vi "SwerveChooseBestAngle.vi"(5 "Goal Override":bool, 7 "Goal Override Angle (deg) [-180,+180]":dbl format="%#_13g", 8 "Hysteresis (deg)":dbl=10.0 format="%#_13g", 10 "Goal Angle (deg) [-180,+180]":dbl format="%#_13g", 11 "Current Angle (deg) [-180,+180]":dbl format="%#_13g") -> (0 "Flip Drive Motor Multiple":dbl, 2 "Angular Distance (deg)":dbl format="%_4g")   [LabVIEW 2020]
doc: "Based on the Current Angle and the Goal Angle, this VI calulates the signed angular distance. Taking into account the option to invert the direction of the swerve drive motor and always picking the shortest travel distance. The hysteresis prevents undesirable vacillation between angle choices."
panel:
  out "Flip Drive Motor Direction":bool
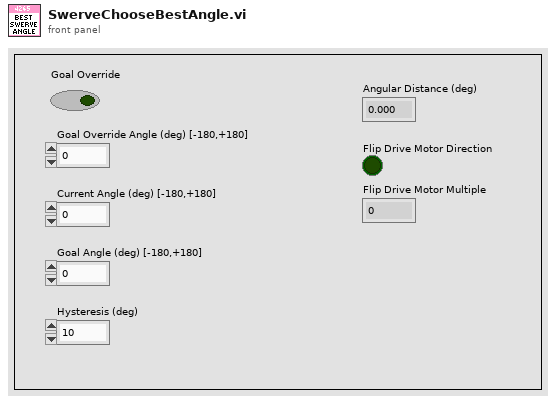
[diagram p1: front panel]
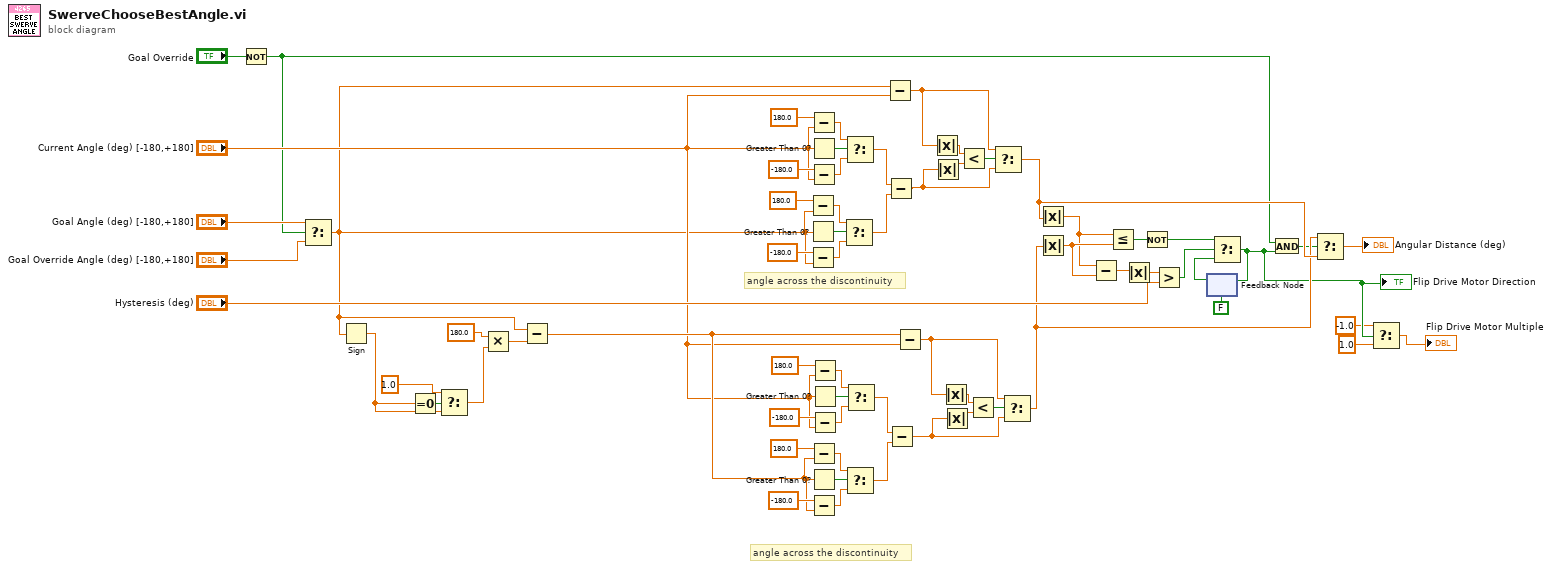
[diagram p0: block diagram]
diagram:
  # "angle across the discontinuity"
  # "angle across the discontinuity"
  n1 = Not(x="Goal Override") -> (.not. x?=w6:bool)
  n2 = Select(t="Goal Angle (deg) [-180,+180]", s=w6, f="Goal Override Angle (deg) [-180,+180]") -> (s? t:f=w8:dbl)
  n3 = Sign(1:w8) -> (0:w16:dbl)
  n4 = Equal To 0?(x=w16) -> (x = 0?=w17:bool)
  n5 = Select(t=1.0, s=w17, f=w16) -> (s? t:f=w13:dbl)
  n6 = Multiply(x=180.0 ("y"), y=w13) -> (x*y=w65:dbl)
  n7 = Subtract(x=w8, y=w65) -> (x-y=w38:dbl)
  n8 = Subtract(x=180.0, y=w8) -> (x-y=w26:dbl)
  n9 = Greater Than 0?(x=w8) -> (x > 0?=w28:bool)
  n10 = Subtract(x=-180.0, y=w8) -> (x-y=w24:dbl)
  n11 = Subtract(x=180.0, y="Current Angle (deg) [-180,+180]") -> (x-y=w31:dbl)
  n12 = Greater Than 0?(x="Current Angle (deg) [-180,+180]") -> (x > 0?=w33:bool)
  n13 = Subtract(x=-180.0, y="Current Angle (deg) [-180,+180]") -> (x-y=w29:dbl)
  n14 = Subtract(x=180.0, y=w38) -> (x-y=w47:dbl)
  n15 = Greater Than 0?(x=w38) -> (x > 0?=w49:bool)
  n16 = Subtract(x=-180.0, y=w38) -> (x-y=w45:dbl)
  n17 = Subtract(x=180.0, y="Current Angle (deg) [-180,+180]") -> (x-y=w53:dbl)
  n18 = Greater Than 0?(x="Current Angle (deg) [-180,+180]") -> (x > 0?=w55:bool)
  n19 = Subtract(x=-180.0, y="Current Angle (deg) [-180,+180]") -> (x-y=w51:dbl)
  n20 = Select(t=w26, s=w28, f=w24) -> (s? t:f=w22:dbl)
  n21 = Select(t=w31, s=w33, f=w29) -> (s? t:f=w23:dbl)
  n22 = Select(t=w47, s=w49, f=w45) -> (s? t:f=w43:dbl)
  n23 = Select(t=w53, s=w55, f=w51) -> (s? t:f=w44:dbl)
  n24 = Subtract(x=w8, y="Current Angle (deg) [-180,+180]") -> (x-y=w34:dbl)
  n25 = Subtract(x=w23, y=w22) -> (x-y=w20:dbl)
  n26 = Subtract(x=w44, y=w43) -> (x-y=w42:dbl)
  n27 = Subtract(x=w38, y="Current Angle (deg) [-180,+180]") -> (x-y=w39:dbl)
  n28 = Absolute Value(x=w34) -> (abs(x)=w35:dbl)
  n29 = Absolute Value(x=w20) -> (abs(x)=w36:dbl)
  n30 = Absolute Value(x=w39) -> (abs(x)=w40:dbl)
  n31 = Absolute Value(x=w42) -> (abs(x)=w41:dbl)
  n32 = Less?(x=w35, y=w36) -> (x < y?=w37:bool)
  n33 = Less?(x=w40, y=w41) -> (x < y?=w50:bool)
  n34 = Select(t=w34, s=w37, f=w20) -> (s? t:f=w12:dbl)
  n35 = Select(t=w39, s=w50, f=w42) -> (s? t:f=w11:dbl)
  n36 = Absolute Value(x=w12) -> (abs(x)=w56:dbl)
  n37 = Absolute Value(x=w11) -> (abs(x)=w57:dbl)
  n38 = Subtract(x=w56, y=w57) -> (x-y=w61:dbl)
  n39 = Less Or Equal?(x=w56, y=w57) -> (x <= y?=w19:bool)
  n40 = Absolute Value(x=w61) -> (abs(x)=w60:dbl)
  n41 = Not(x=w19) -> (.not. x?=w18:bool)
  n42 = Greater?(x=w60, y="Hysteresis (deg)") -> (0:w58:bool)
  n43 = feedback #1(FALSE) -> (w63:bool)
  n44 = Select(t=w18, s=w58, f=w63) -> (s? t:f=w4:bool)
  "Flip Drive Motor Direction" <- w4
  n45 = feedback-in #1(w4) -> ()
  n46 = And(x=w6, y=w4) -> (x .and. y?=w10:bool)
  n47 = Select(t=w11, s=w10, f=w12) -> (s? t:f=→"Angular Distance (deg)":dbl)
  n48 = Select(t=-1.0, s=w4, f=1.0) -> (s? t:f=→"Flip Drive Motor Multiple":dbl)
